vi "encode-to-json-cdaq.vi"(8 "Sensor Options":T1={"Display Units"="units", "Zero Offset"=2.62, "Sensor Min"=0.0, "Sensor Max"=500.0, "Signal Min"=0.0, "Signal Max"=100.0, "Conversion Factor"=0.0}, 10 "Datalogging options":T2={"data-precision"=3, "Include Date"=FALSE, "Include Timestamp"=TRUE, "Include Milliseconds"=FALSE, "sample-rate (Hz)"=4.0, "Logging Active"=TRUE}, 11 "Filepath Selection":T3={"Log Filepath Source"=enum."Application Relative (Auto)", "Log File Path (Manual)"=path "C:/Users/dheard/Documents/0002-labview-projects/ammonia-absorbsion-rig/data", "Log File Folder Name"="data", "log file name"="log", "Include Date in Filename"=TRUE, "Include Time in Filename"=TRUE}) -> (0 "sensor-options-json":string, 2 "data-logging-json":string, 3 "filepath-json":string)   [LabVIEW 2024]
uses:
  utils-sub-vi/csv-file-logging-util/filepath-selection.ctl
  utils-sub-vi/csv-file-logging-util/datalogging-options.ctl
  sensor-options.ctl
  filepath-json-cluster-feck.ctl
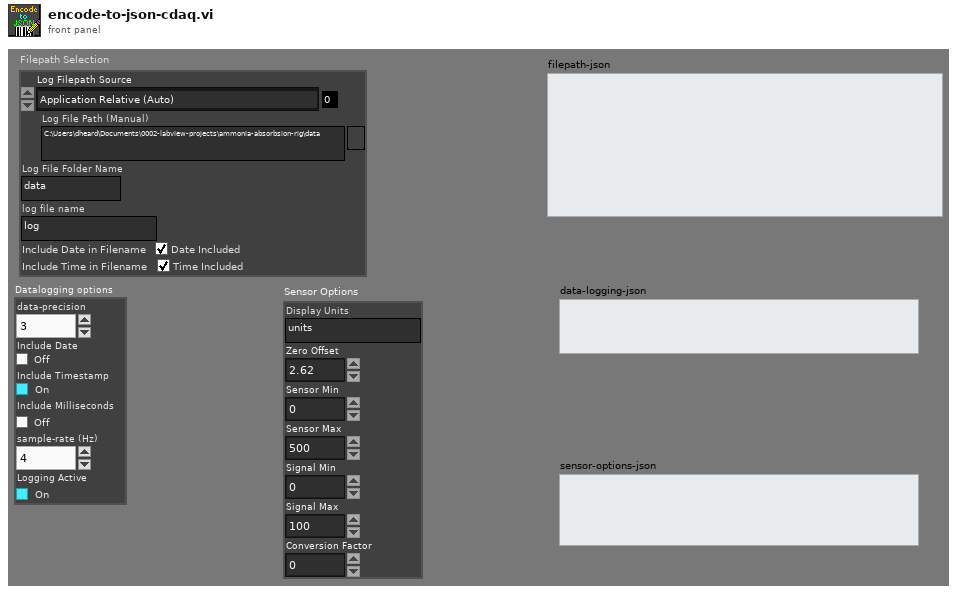
[diagram p1: front panel]
types:
  T1 = typedef "sensor-options.ctl" = cluster{"Display Units":string, "Zero Offset":dbl, "Sensor Min":dbl, "Sensor Max":dbl, "Signal Min":dbl, "Signal Max":dbl, "Conversion Factor":dbl}
  T2 = typedef "datalogging-options.ctl" = cluster{"data-precision":i32, "Include Date":bool, "Include Timestamp":bool, "Include Milliseconds":bool, "sample-rate (Hz)":dbl, "Logging Active":bool}
  T3 = typedef "filepath-selection.ctl" = cluster{"Log Filepath Source":enum16{"Application Relative (Auto)", "VI Relative (Auto)", "Complete Path (Manual)"}, "Log File Path (Manual)":path, "Log File Folder Name":string, "log file name":string, "Include Date in Filename":bool, "Include Time in Filename":bool}
  T4 = typedef "filepath-json-cluster-feck.ctl" = cluster{"Log Filepath Source":i32, "Log Filepath byte array":u8[], "Log File Folder Name":string, "log file name":string, "Include Date in Filename":bool, "Include Time in Filename":bool}
  T5 = enum16{"Application Relative (Auto)", "VI Relative (Auto)", "Complete Path (Manual)"}
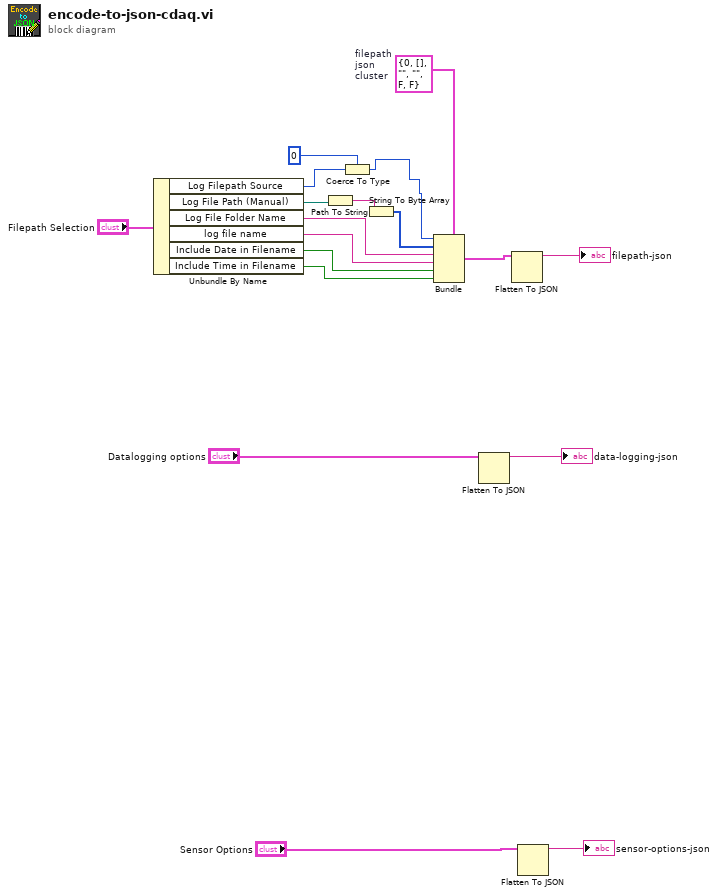
[diagram p0: block diagram]
diagram:
  w4 = T4 {"Log Filepath Source"=0, "Log Filepath byte array"=[], "Log File Folder Name"="", "log file name"="", "Include Date in Filename"=FALSE, "Include Time in Filename"=FALSE}  # filepath json cluster
  n1 = Unbundle By Name("Filepath Selection") -> ("Log Filepath Source"=w6:T5, "Log File Path (Manual)"=w5:path, "Log File Folder Name"=w18:string, "log file name"=w17:string, "Include Date in Filename"=w16:bool, "Include Time in Filename"=w15:bool)
  n2 = Path To String(path=w5) -> (string=w10:string)
  n3 = Coerce To Type(0:w6, 1:0) -> (2:w2:i32)
  n4 = String To Byte Array(string=w10) -> (unsigned byte array=w9:u8[])
  n5 = Bundle(cluster=w4, "Log Filepath Source"=w2, "Log Filepath byte array"=w9, "Log File Folder Name"=w18, "log file name"=w17, "Include Date in Filename"=w16, "Include Time in Filename"=w15) -> (w3:T4)
  n6 = Flatten To JSON(anything="Datalogging options") -> (JSON string=→"data-logging-json":string)  [unwired: 2 in, 1 out]
  n7 = Flatten To JSON(anything=w3) -> (JSON string=→"filepath-json":string)  [unwired: 2 in, 1 out]
  n8 = Flatten To JSON(anything="Sensor Options") -> (JSON string=→"sensor-options-json":string)  [unwired: 2 in, 1 out]
